vi "Self Configure.vi"(8 "error in":errorcluster, 11 "Analog-Output in":refnum<class "Analog-Output.lvclass">) -> (0 "error out":errorcluster, 3 "Analog-Output out":refnum<class "Analog-Output.lvclass">)   [LabVIEW 2019, in "Analog-Output.lvlib" / "Analog-Output.lvclass"]
doc: "Children of Instruments must override this routine and call the parent method. \nThis routine is implemented to allow each instrument to read its specific configuration keys and implement any default configuration settings.\n\nThis routine already calls Connect and Self Test Routines."
uses:
  Library/Analog-Output.lvclass
  Custom Controls/Configuration Keys.ctl
  Library/Analog-Output.lvclass/Analog-Output.ctl
  builds/Instruments/Instruments.lvlibp/Library/Instruments.lvclass
  builds/Tools/Config.lvlibp/Config.lvclass
  C:/Users/Public/Documents/Development/builds/Tools/Config.lvlibp/Config.lvclass
panel:
  in  "Configuration Keys":T1
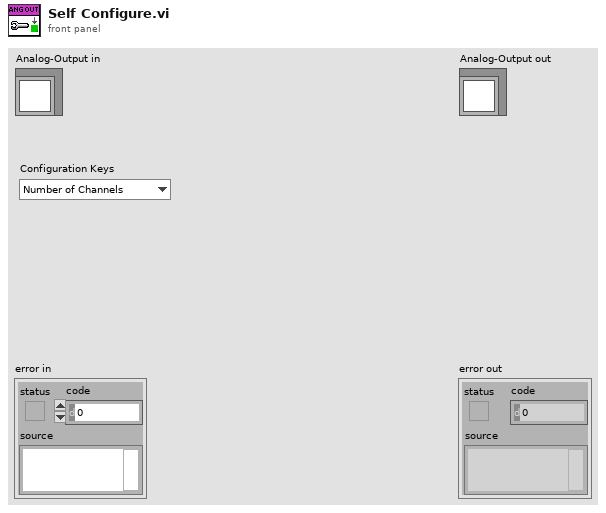
[diagram p1: front panel]
types:
  T1 = typedef "Analog-Output.lvlib/Analog-Output.lvclass/Configuration Keys.ctl" = enum16{"Number of Channels"}
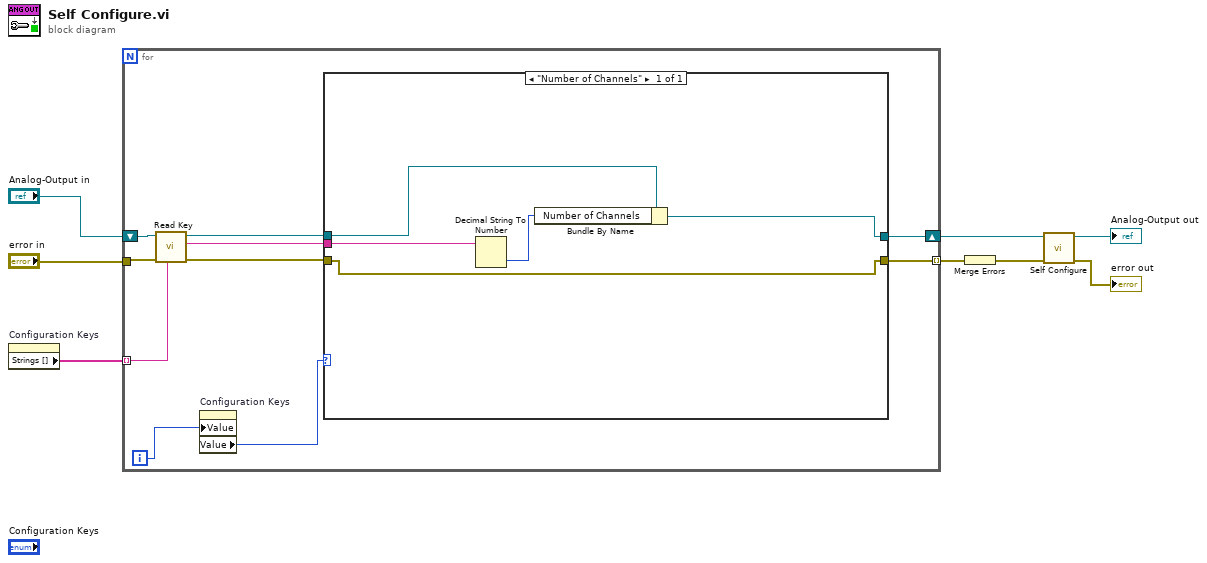
[diagram p0: block diagram]
diagram:
  n1 = property on="Configuration Keys" class="Enum (strict)"() -> ("Strings []"=w5:string[])  [unwired: 2 in, 2 out]
  n2 = for {
    tunnel: "error in" -> [w14]
    tunnel: w5 -> [w18] mode=indexing
    shift-right: [w12] -> w3
    shift-left: "Analog-Output in" -> [w17]
    tunnel: [w11] -> w1 mode=indexing
    i -> [w10]
    n3 = call "Read Key.vi"("Key Name"=w18, "error in"=w14, "Config in"=w17) -> ("error out"=w13:errorcluster, "Key Value"=w15:string, "Config out"=w16:refnum<class "Analog-Output.lvclass">)  [unwired: 6 in]
    n4 = property on="Configuration Keys" class="Enum (strict)"("Value"=w10) -> ("Value"=w9:T1)  [unwired: 2 in, 2 out]
    n5 = case shown="\"Number of Channels\"" w9 {
      tunnel: w16 -> [w22]
      tunnel: w15 -> [w23]
      tunnel: w13 -> [w19]
      tunnel: [w20] -> w12
      tunnel: [w19] -> w11
      frame "Number of Channels" {
        n6 = Decimal String To Number(string=w23) -> (number=w21:i32)  [unwired: 2 in, 1 out]
        n7 = Bundle By Name(cluster=w22, "Number of Channels"=w21) -> (w20:refnum<class "Analog-Output.lvclass">)
      }
    }
  }
  n8 = Merge Errors(w1) -> (w2:errorcluster)
  n9 = call-parent "Self Configure.vi"("error in"=w2, "Instruments in"=w3) -> ("error out"=→"error out":errorcluster, "Instruments out"=→"Analog-Output out":refnum<class "Analog-Output.lvclass">)  [unwired: 8 in]
